vi "!How to Use Progress Bar.vi"   [LabVIEW 2019]
panel:
  # "Run Me!"
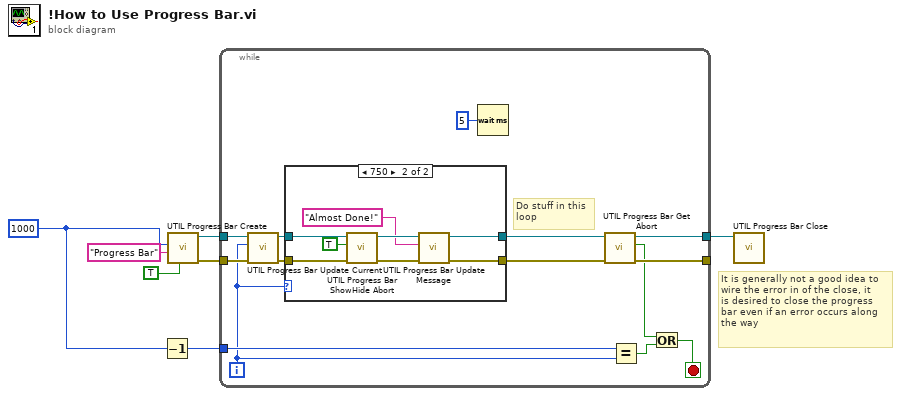
[diagram p0: block diagram]
diagram:
  w2 = 1000 ("High")
  # "It is generally not a good idea to\nwire the error in of the close, it\nis desired to close the progress\nbar even if an error occurs along\nthe way"
  n1 = Decrement(x=w2) -> (x-1=w1:i32)
  n2 = call "UTIL Progress Bar Create.vi"("Show Progress Bar"=TRUE, "Message"="Progress Bar", "High"=w2) -> ("error out"=w6:errorcluster, "reference"=w7:refnum<vi>)  [unwired: 7 in]
  n3 = while {
    tunnel: w7 -> [w20]
    tunnel: w6 -> [w21]
    tunnel: [w15] -> _
    tunnel: [w14] -> w3
    tunnel: w1 -> [w11]
    i -> [w10]
    stop <- w9 stop-if-true
    # "Do stuff in this\nloop"
    n4 = call "UTIL Progress Bar Update Current.vi"("error in (no error)"=w21, "Current"=w10, "reference in"=w20) -> ("error out"=w19:errorcluster, "reference out"=w18:refnum<vi>)  [unwired: 7 in]
    n5 = case shown="750" w10 {
      tunnel: w19 -> [w22 w31]
      tunnel: w18 -> [w23 w29]
      tunnel: [w22 w25] -> w17
      tunnel: [w23 w24] -> w16
      frame Default {
      }
      frame 750 {
        n6 = call "UTIL Progress Bar ShowHide Abort.vi"("error in (no error)"=w31, "Show Abort"=TRUE, "reference in"=w29) -> ("error out"=w28:errorcluster, "reference out"=w27:refnum<vi>)  [unwired: 7 in]
        n7 = call "UTIL Progress Bar Update Message.vi"("error in (no error)"=w28, "Message"="Almost Done!", "reference in"=w27) -> ("error out"=w25:errorcluster, "reference out"=w24:refnum<vi>)  [unwired: 7 in]
      }
    }
    n8 = Wait (ms)(milliseconds to wait=u32 5) -> ()  [unwired: 1 out]
    n9 = call "UTIL Progress Bar Get Abort.vi"("error in (no error)"=w17, "reference in"=w16) -> ("error out"=w15:errorcluster, "Abort"=w13:bool, "reference out"=w14:refnum<vi>)  [unwired: 7 in]
    n10 = Equal?(x=w11, y=w10) -> (x = y?=w12:bool)
    n11 = Or(x=w13, y=w12) -> (x .or. y?=w9:bool)
  }
  n12 = call "UTIL Progress Bar Close.vi"("reference in"=w3) -> ()  [unwired: 10 in, 1 out]
